vi "Set_ADCQuality.vi"(8 "error in":errorcluster, 10 "PicamAdcQuality":T1=1 items=["LowNoise"=1, "HighCapacity"=2, "ElectronMultiplied"=3, "HighSpeed"=4], 11 "camera handle in":u64) -> (0 "error out":errorcluster, 3 "camera handle out":u64)   [LabVIEW 2019, in "PICam.lvlib"]
doc: "PicamAdcQuality is the set of Analog-to-Digital conversion techniques and quality settings\nfor pixel digitization.\n\nPicamAdcQuality_LowNoise Optimized for the lowest noise.\nPicamAdcQuality_HighCapacity Optimized for sensing high levels of radiation.\nPicamAdcQuality_ElectronMultiplied Provides electron multiplication.\n\nWarning: the \"HighSpeed\" mode is not applicable for PIXIS (and maybe some other) cams!"
uses:
  PICam.lvlib
  Ctrls/PicamAdcQuality.ctl
  Picam64.dll   
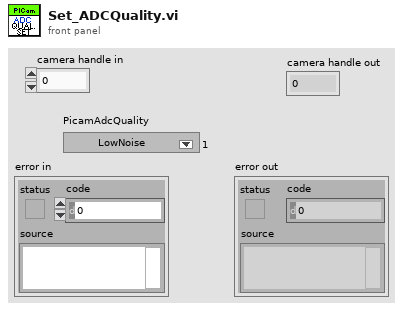
[diagram p1: front panel]
types:
  T1 = typedef "PICam.lvlib/PicamAdcQuality.ctl" = u32
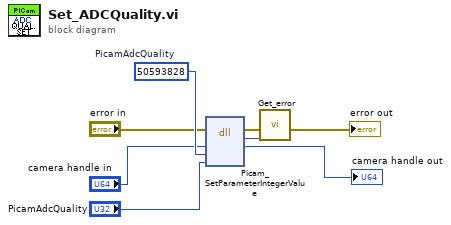
[diagram p0: block diagram]
diagram:
  w4 = u32 50593828  # PicamAdcQuality
  n1 = dll-call lib="Picam32.dll" fn="Picam_SetParameterIntegerValue"(error in="error in", "camera"="camera handle in", "PicamParameter"=w4, "PicamAdcQuality"="PicamAdcQuality") -> (error out=w8:errorcluster, "return type"=w7:i32, "camera"=→"camera handle out":u64)  [unwired: 4 in, 1 out]
  n2 = call "Get_error.vi"("PICam_Error"=w7, "error in (no error)"=w8) -> ("error out"=→"error out":errorcluster)  [unwired: 9 in]
